vi "util_camSnapImageTest.vi"() -> ()   [LabVIEW 2013]
uses:
  <vilib>/vision/driver/NI_Vision_Acquisition_Software.lvlib
panel:
  in  "Interface Name":string="cam0"
  out "error out":errorcluster
  in  "error in":errorcluster
  out "Image Out":T1(plugin-control)
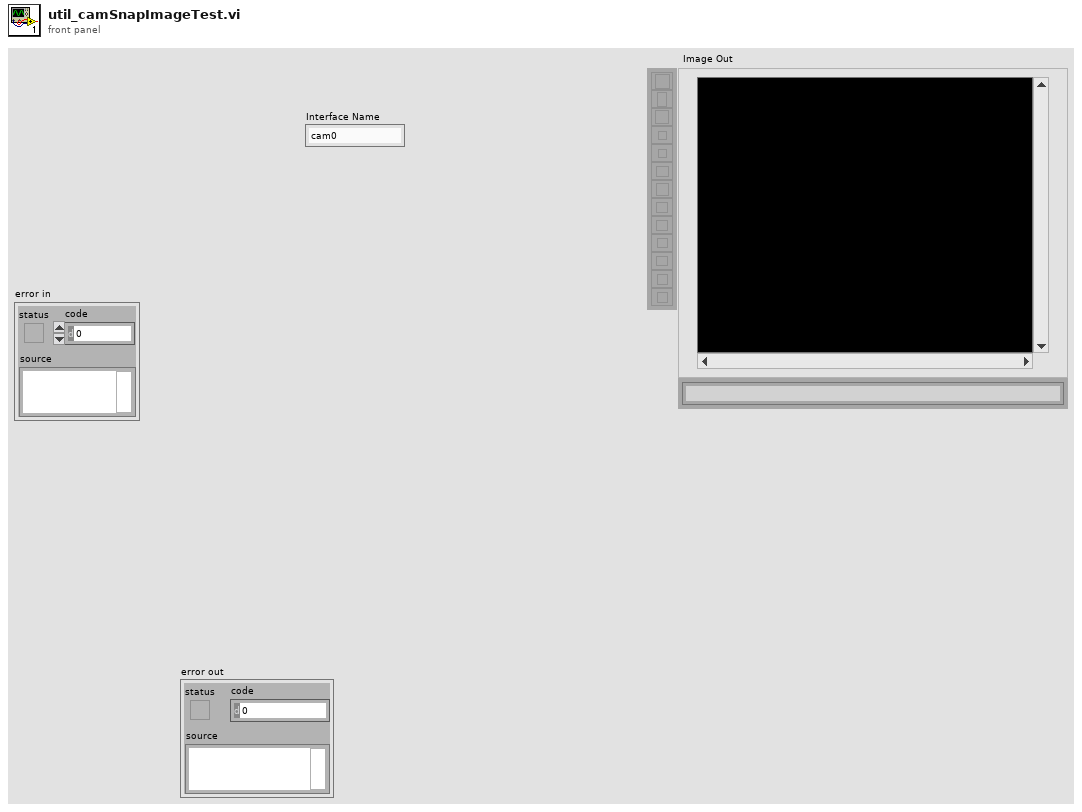
[diagram p1: front panel]
types:
  T1 = typedef "IMAQ Image.ctl" = refnum<image>
  T2 = typedef "IMAQdx.ctl" = refnum<k21>
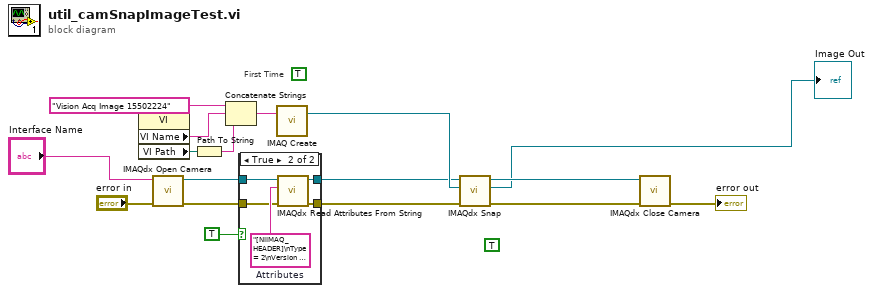
[diagram p0: block diagram]
diagram:
  (unwired) TRUE
  (unwired) TRUE
  # "First Time"
  n1 = property class="VI"() -> ("VI Name"=w14:string, "VI Path"=w15:path)  [unwired: 2 in, 2 out]
  n2 = call <vilib>:"IMAQdx Open Camera.vi"("error in"="error in", "Session In"="Interface Name") -> ("error out"=w9:errorcluster, "Session Out"=w10:T2)  [unwired: 1 in, 7 out]
  n3 = Path To String(path=w15) -> (string=w13:string)
  n4 = Concatenate Strings("Vision Acq Image 15502224" ("Image Name"), w14, w13) -> (w11:string)
  n5 = case shown="True" TRUE ("Init Attributes") {
    tunnel: w10 -> [w19 w24]
    tunnel: w9 -> [w18 w22]
    tunnel: [w19 w21] -> w4
    tunnel: [w18 w20] -> w8
    frame False {
    }
    frame True {
      w23 = "[NIIMAQ_HEADER]\nType = 2\nVersion = 8\n\n[CAMERA_DATA]\nAcquisitionAttributes::Bayer::Algorithm = \"Bilinear\"\nAcquisitionAttributes::Bayer::GainB = \"1\"\nAcquisitionAttributes::Bayer::GainG = \"1\"\nAcquisitionAttributes::Bayer::GainR = \"1\"\nAcquisitionAttributes::Bayer::Pattern = \"Use hardware value\"\nAcquisitionAttributes::BitsPerPixel = \"Use hardware value\"\nAcquisitionAttributes::IgnoreFirstFrame = \"false\"\nAcquisitionAttributes::ImageDecoderCopyMode = \"Auto\"\nAcquisitionAttributes::OutputImageType = \"Auto\"\nAcquisitionAttributes::OverwriteMode = \"Get Newest\"\nAcquisitionAttributes::PixelSignedness = \"Use hardware value\"\nAcquisitionAttributes::ReceiveTimestampMode = \"None\"\nAcquisitionAttributes::ShiftPixelBits = \"false\"\nAcquisitionAttributes::SwapPixelBytes = \"false\"\nAcquisitionAttributes::Timeout = \"5000\"\nAcquisitionAttributes::VerticalMirror = \"false\"\nAcquisitionAttributes::VideoMode = \"1280x800 RGB24 10.00fps\"\nCameraAttributes::BacklightCompensation::Mode = \"Manual\"\nCameraAttributes::BacklightCompensation::Value = \"false\"\nCameraAttributes::Brightness::Mode = \"Manual\"\nCameraAttributes::Brightness::Value = \"133\"\nCameraAttributes::Contrast::Mode = \"Manual\"\nCameraAttributes::Contrast::Value = \"0.050000000000000003\"\nCameraAttributes::Exposure::Mode = \"Auto\"\nCameraAttributes::Pan::Mode = \"Manual\"\nCameraAttributes::Pan::Value = \"0\"\nCameraAttributes::Saturation::Mode = \"Manual\"\nCameraAttributes::Saturation::Value = \"83\"\nCameraAttributes::Sharpness::Mode = \"Manual\"\nCameraAttributes::Sharpness::Value = \"25\"\nCameraAttributes::Tilt::Mode = \"Manual\"\nCameraAttributes::Tilt::Value = \"0\"\nCameraAttributes::WhiteBalance::Mode = \"Auto\"\nCameraAttributes::Zoom::Mode = \"Manual\"\nCameraAttributes::Zoom::Value = \"0\"\n"  # Attributes
      n6 = call <vilib>:"IMAQdx Read Attributes From String.vi"("error in"=w22, "Attributes String In"=w23, "Session In"=w24) -> ("error out"=w20:errorcluster, "Session Out"=w21:T2)  [unwired: 7 out]
    }
  }
  n7 = call "IMAQ Create"("Image Name"=w11) -> ("New Image"=w5:T1)  [unwired: 3 in, 2 out]
  n8 = call <vilib>:"IMAQdx Snap.vi"("error in"=w8, "Image In"=w5, "Session In"=w4) -> ("error out"=w6:errorcluster, "Image Out"=→"Image Out":T1, "Session Out"=w2:T2)  [unwired: 6 out]
  n9 = call <vilib>:"IMAQdx Close Camera.vi"("error in"=w6, "Session In"=w2) -> ("error out"=→"error out":errorcluster)  [unwired: 9 out]
